vi "Teleop.vi"(10 "Match Info":T1={"Autonomous Elapsed Seconds"=0.0, "TeleOp Elapsed Seconds"=0.0, "Disabled Elapsed Seconds"=0.0, "Visited Autonomous"=FALSE, "Visited TeleOp"=FALSE, "Visited Disabled"=FALSE, "Autonomous Settings"={"Autonomous Style"=enum."Independent", "VI Refnum"=refnum}}, 11 "Call Context":T2) -> ()   [LabVIEW 2019]
doc: "This VI is called for each TeleOp packet received from the DS where the robot is not disabled. It is often used to read from the joysticks and update I/O or to update setpoints for timed control loops. It should complete and return within 20 milliseconds or it may miss DS packets."
uses:
  <vilib>/Rock Robotics/WPI/DriverStation/WPI_DriverStationDerivedRobotMode.ctl
  <vilib>/Rock Robotics/WPI/DriverStation/WPI_DriverStationMatch Info.ctl
  <vilib>/Rock Robotics/WPI/Utilities/WPI_GetSetVariantRefNum.vi
  JoysticksGlobal.vi
  <vilib>/Rock Robotics/Network Tables/NT Read Boolean.vi
  <vilib>/Rock Robotics/Network Tables/NT Read Number.vi
panel:
  out "Sample Slider 0":dbl(slide) scale=0.0..5.0
  out "Sample Boolean 1":bool
  out "Sample Boolean 0":bool
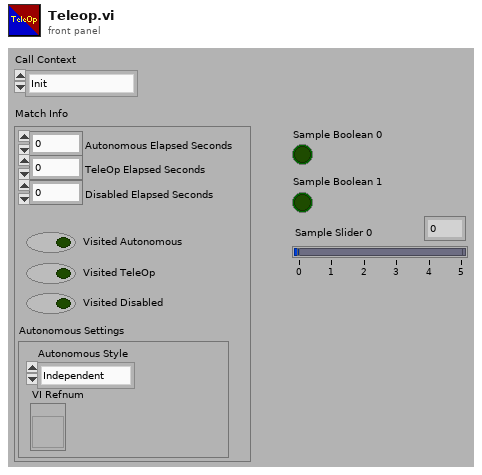
[diagram p1: front panel]
types:
  T1 = typedef "WPI_DriverStationMatch Info.ctl" = cluster{"Autonomous Elapsed Seconds":dbl, "TeleOp Elapsed Seconds":dbl, "Disabled Elapsed Seconds":dbl, "Visited Autonomous":bool, "Visited TeleOp":bool, "Visited Disabled":bool, "Autonomous Settings":cluster{"Autonomous Style":enum16{"Iterative", "Independent"}, "VI Refnum":refnum<vi>}}
  T2 = typedef "WPI_DriverStationDerivedRobotMode.ctl" = enum16{"Init", "Execute", "Stop"}
  T3 = typedef "WPI_JoystickDevRef.ctl" = cluster{"Device":T4}
  T4 = typedef "WPI_JoystickDeviceEnum.ctl" = enum16{"USB 0", "USB 1", "USB 2", "USB 3", "USB 4", "USB 5"}
  T5 = typedef "D-Pad.ctl" = cluster{"Top":bool, "Bottom":bool, "None":bool, "Right":bool, "Left":bool}
  T6 = typedef "Button Cluster.ctl" = cluster{"Buttons[0]":bool, "Buttons[1]":bool, "Buttons[2]":bool, "Buttons[3]":bool, "Buttons[4]":bool, "Buttons[5]":bool, "Buttons[6]":bool, "Buttons[7]":bool, "Buttons[8]":bool, "Buttons[9]":bool}
  T7 = typedef "Axes Cluster.ctl" = cluster{"Axes[0]":dbl, "Axes[1]":dbl, "Axes[2]":dbl, "Axes[3]":dbl, "Axes[4]":dbl, "Axes[5]":dbl, "Axes[6]":dbl, "Axes[7]":dbl, "Axes[8]":dbl}
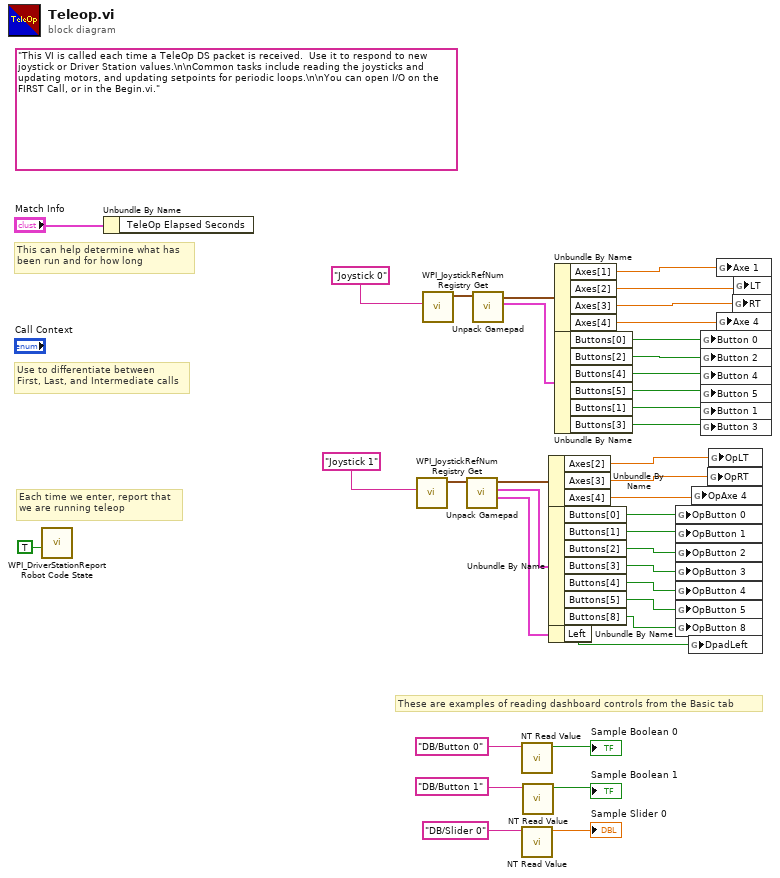
[diagram p0: block diagram]
diagram:
  (unwired) "This VI is called each time a TeleOp DS packet is received.  Use it to respond to new joystick or Driver Station values.\n\nCommon tasks include reading the joysticks and updating motors, and updating setpoints for periodic loops.\n\nYou can open I/O on the FIRST Call, or in the Begin.vi."
  # "These are examples of reading dashboard controls from the Basic tab"
  # "Each time we enter, report that\nwe are running teleop"
  # "Use to differentiate between\nFirst, Last, and Intermediate calls"
  # "This can help determine what has\nbeen run and for how long"
  n1 = call <vilib>:"WPI_DriverStationReport Robot Code State.vi"("TeleOp"=TRUE ("Autonomous")) -> ()  [unwired: 10 in, 1 out]
  n2 = Unbundle By Name("Match Info") -> ()  [unwired: 1 out]
  n3 = call <vilib>:"WPI_JoystickRefNum Registry Get.vi"("refnum name"="Joystick 1") -> ("JoystickDevRef"=w19:T3)  [unwired: 1 in, 9 out]
  n4 = call <vilib>:"WPI_JoystickRefNum Registry Get.vi"("refnum name"="Joystick 0") -> ("JoystickDevRef"=w28:T3)  [unwired: 1 in, 9 out]
  n5 = call "Unpack Gamepad.vi"("JoystickDevRef"=w19) -> ("D-Pad"=w14:T5, "Button Cluster"=w17:T6, "Axes"=w18:T7)  [unwired: 8 in]
  n6 = call "Unpack Gamepad.vi"("JoystickDevRef"=w28) -> ("Button Cluster"=w26:T6, "Axes"=w27:T7)  [unwired: 8 in, 1 out]
  n7 = call-poly <vilib>:"NT Read Value.vi"("Name"="DB/Button 0" ("refnum name")) -> ("Boolean"=→"Sample Boolean 0":bool)  [unwired: 9 in, 1 out]
  n8 = call-poly <vilib>:"NT Read Value.vi"("Name"="DB/Slider 0" ("refnum name")) -> ("Numeric"=→"Sample Slider 0":dbl)  [unwired: 9 in, 1 out]
  n9 = call-poly <vilib>:"NT Read Value.vi"("Name"="DB/Button 1" ("refnum name")) -> ("Boolean"=→"Sample Boolean 1":bool)  [unwired: 9 in, 1 out]
  n10 = Unbundle By Name(w18) -> ("Axes[2]"=w16:dbl, "Axes[3]"=w15:dbl, "Axes[4]"=w6:dbl)
  n11 = Unbundle By Name(w17) -> ("Buttons[0]"=w13:bool, "Buttons[1]"=w7:bool, "Buttons[2]"=w8:bool, "Buttons[3]"=w9:bool, "Buttons[4]"=w10:bool, "Buttons[5]"=w11:bool, "Buttons[8]"=w3:bool)
  n12 = Unbundle By Name(w14) -> ("Left"=w12:bool)
  n13 = Unbundle By Name(w27) -> ("Axes[1]"=w25:dbl, "Axes[2]"=w24:dbl, "Axes[3]"=w23:dbl, "Axes[4]"=w22:dbl)
  n14 = Unbundle By Name(w26) -> ("Buttons[0]"=w21:bool, "Buttons[2]"=w20:bool, "Buttons[4]"=w5:bool, "Buttons[5]"=w4:bool, "Buttons[1]"=w2:bool, "Buttons[3]"=w1:bool)
  n15 = global write "JoysticksGlobal.vi" "OpButton 0"(w13) -> ()
  n16 = global write "JoysticksGlobal.vi" "OpButton 1"(w7) -> ()
  n17 = global write "JoysticksGlobal.vi" "OpButton 2"(w8) -> ()
  n18 = global write "JoysticksGlobal.vi" "OpButton 3"(w9) -> ()
  n19 = global write "JoysticksGlobal.vi" "OpButton 4"(w10) -> ()
  n20 = global write "JoysticksGlobal.vi" "OpButton 5"(w11) -> ()
  n21 = global write "JoysticksGlobal.vi" "OpButton 8"(w3) -> ()
  n22 = global write "JoysticksGlobal.vi" "DpadLeft"(w12) -> ()
  n23 = global write "JoysticksGlobal.vi" "OpAxe 4"(w6) -> ()
  n24 = global write "JoysticksGlobal.vi" "Button 0"(w21) -> ()
  n25 = global write "JoysticksGlobal.vi" "Button 2"(w20) -> ()
  n26 = global write "JoysticksGlobal.vi" "Button 4"(w5) -> ()
  n27 = global write "JoysticksGlobal.vi" "Button 5"(w4) -> ()
  n28 = global write "JoysticksGlobal.vi" "Button 1"(w2) -> ()
  n29 = global write "JoysticksGlobal.vi" "Button 3"(w1) -> ()
  n30 = global write "JoysticksGlobal.vi" "OpRT"(w15) -> ()
  n31 = global write "JoysticksGlobal.vi" "OpLT"(w16) -> ()
  n32 = global write "JoysticksGlobal.vi" "Axe 1"(w25) -> ()
  n33 = global write "JoysticksGlobal.vi" "Axe 4"(w22) -> ()
  n34 = global write "JoysticksGlobal.vi" "RT"(w23) -> ()
  n35 = global write "JoysticksGlobal.vi" "LT"(w24) -> ()
